vi "Ignore.vi"(8 "error in (no error)":errorcluster, 11 "JSON Lexer in":refnum<class "JSON Lexer.lvclass">) -> (0 "error out":errorcluster, 3 "JSON Lexer out":refnum<class "JSON Lexer.lvclass">)   [LabVIEW 2013, in "JKI JSON Serialization.lvlib" / "JSON Lexer.lvclass"]
uses:
  JSON Lexer.lvclass
  JSON Lexer.lvclass/JSON Lexer.ctl
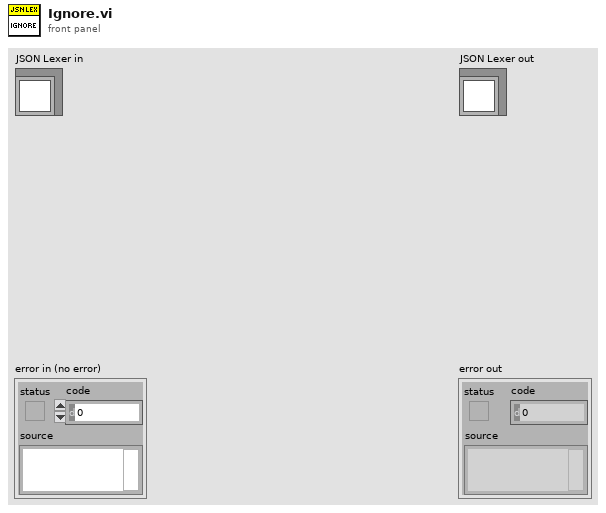
[diagram p1: front panel]
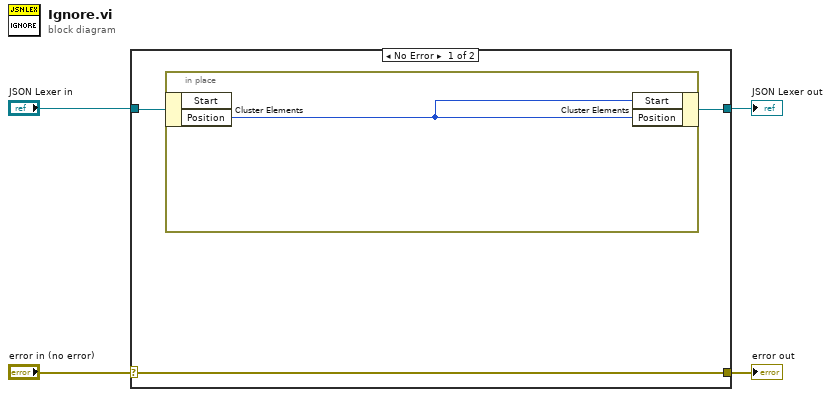
[diagram p0: block diagram]
diagram:
  n1 = case shown="No Error" "error in (no error)" {
    selector: "error in (no error)" -> [w7 w10]
    tunnel: [w7 w10] -> w3
    tunnel: [w5 w9] -> w1
    tunnel: "JSON Lexer in" -> [w6 w9]
    frame No Error {
      n2 = in-place {
        n3 = in-place-cluster #1(w6) -> ("Position"=w8:i32)  [unwired: 1 out]
        n4 = in-place-cluster #1("Start"=w8, "Position"=w8) -> (w5:refnum<class "JSON Lexer.lvclass">)
      }
    }
    frame Error {
    }
  }
  "error out" <- w3
  "JSON Lexer out" <- w1
